vi "Main.vi"() -> ()   [LabVIEW 2018]
doc: "Cet exemple de projet Mesure continue est basé sur le modèle Gestionnaire de messages dans une file d'attente.\n\nLa boucle de gestion d'événements génère des messages en fonction des actions sur l'interface utilisateur.\n\nLa boucle de gestion de messages traite les messages générés par la boucle de gestion d'événements ou par d'autres messages. Il y a aussi des sous-VIs de boucle de gestion de messages d'acquisition et d'enregistrement, ainsi qu'une boucle de mise à jour du graphe déroulant."
uses:
  Settings/Settings.ctl
  Acquisition/Hardware Configuration.ctl
  Acquisition/Signal Type.ctl
  Logging/Logging Configuration.ctl
  controls/UI Data.ctl
  controls/UI State.ctl
  support/Message Queue/Enqueue Message (Single).vi
  support/Message Queue/Enqueue Message (Array).vi
  <vilib>/Utility/error.llb/Error Cluster From Error Code.vi
  <vilib>/ErrorRing/Error Ring.xnode
  Acquisition/Acquisition.lvlib
  Logging/Logging.lvlib
  Settings/Settings.lvlib
  support/User Event - Stop/User Event - Stop.lvlib
  support/Message Queue/Message Queue.lvlib
  Settings/Settings Dialog.vi
panel:
  in  "Panneaux":enum32{"MAPA Tech"}(tab)
  out "Graphe d'intensité":dbl[][](graph)
  out "Booléen":bool
  out "Longueur d'onde":dbl
  out "Puissance":dbl
  out "Puissance prédite":dbl
  out "Longueur d'onde":dbl(knob) scale=550.0..2550.0
  out "Puissance prédite":dbl(knob) scale=0.0..10.0
  out "Puissance":dbl(knob) scale=0.0..10.0
  in  "Param status":bool
  out "Données":waveform(dbl)[](graph)
  out "État":string
  in  "Quitter":bool
  in  "Arrêter":bool
  in  "Démarrer":bool
  in  "Paramètres":bool
  # "MAPA Tech"
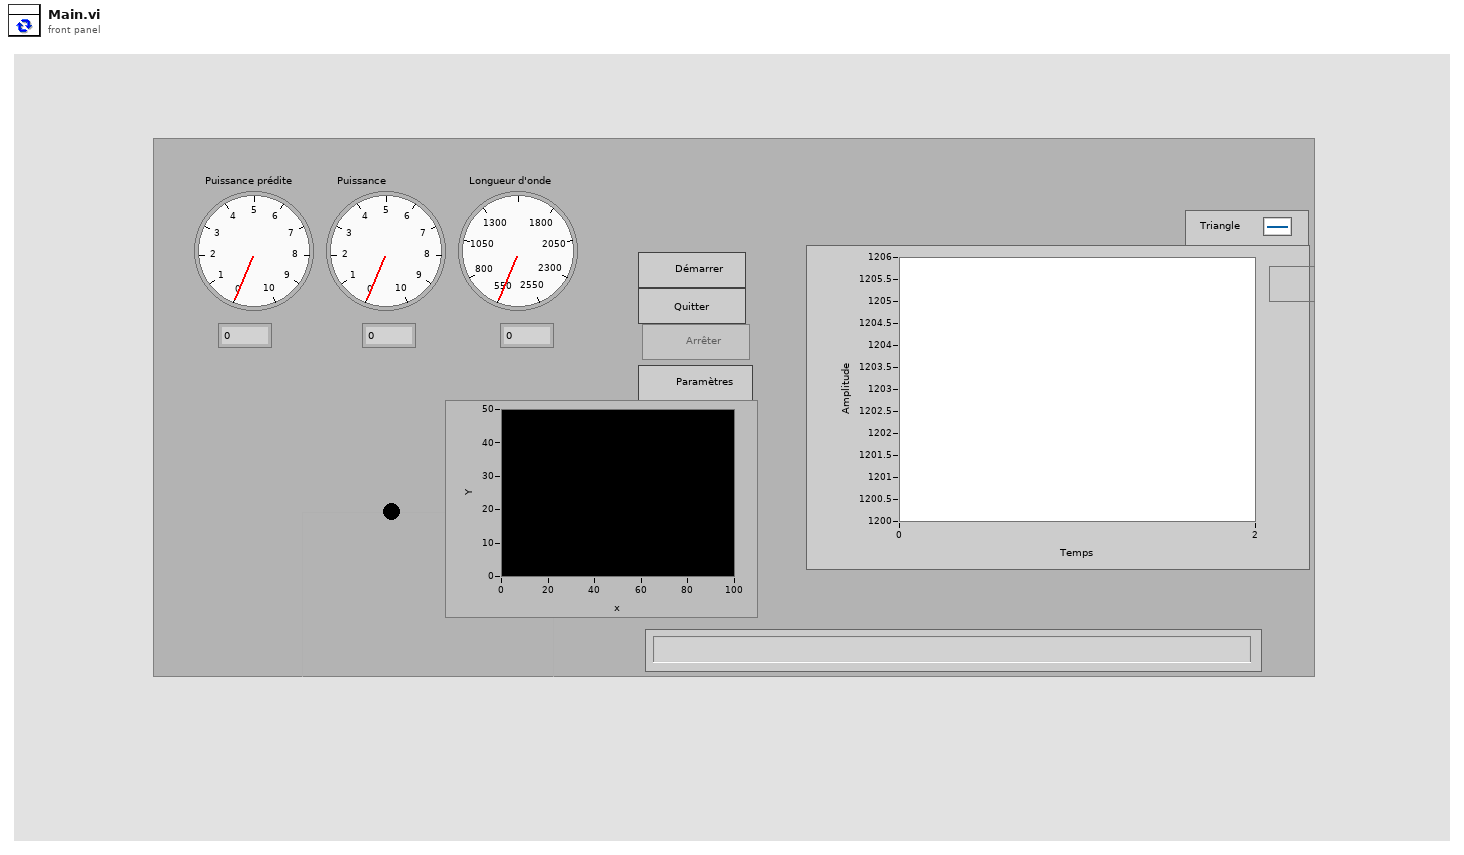
[diagram p1: front panel]
types:
  T1 = typedef "UI State.ctl" = enum16{"Idle", "Acquiring and Logging", "Waiting for Exit", "Waiting for Exit (Acq Stopped)", "Waiting for Exit (Log Stopped)", "Waiting for Stop", "Waiting for Stop (Acq Stopped)", "Waiting for Stop (Log Stopped)"}
  T2 = typedef "UI Data.ctl" = cluster{"Réf. de Démarrer":refnum<vi>, "Réf. d'Arrêter":refnum<vi>, "Réf. de Paramètres":refnum<vi>, "Réf. de Quitter":refnum<vi>, "Réf. d'état":refnum<vi>, "Réf. de données":refnum<vi>, "Ref. Moyennage sélectionneur":refnum<vi>, "Ref. Param status":refnum<vi>}
  T3 = typedef "Settings.lvlib/Settings.ctl" = cluster{"Configuration du matériel":T4, "Configuration de l'enregistrement":T6, "Commande numérique":dbl}
  T4 = typedef "Acquisition.lvlib/Hardware Configuration.ctl" = cluster{"Refnum de matériel <À remplacer>":string, "Type de signal <À remplacer>":T5, "Choix de la longueur d'onde":dbl, "Nom du périphérique":tag, "Choix mode":bool}
  T5 = typedef "Acquisition.lvlib/Signal Type.ctl" = enum16{"Sine Wave", "Square with Noise", "Signal triangulaire", "Simulation DAQ"}
  T6 = typedef "Logging.lvlib/Logging Configuration.ctl" = cluster{"Chemin de base du fichier journal":path, "Référence de fichier TDMS":refnum<k34>}
  T7 = cluster{"état":bool, "code":i32, "source":string}
  T8 = typedef "Message Queue.lvlib/All Message Queues.ctl" = cluster{"IU":refnum<queue>, "Acquisition":refnum<queue>, "Enregistrement":refnum<queue>}
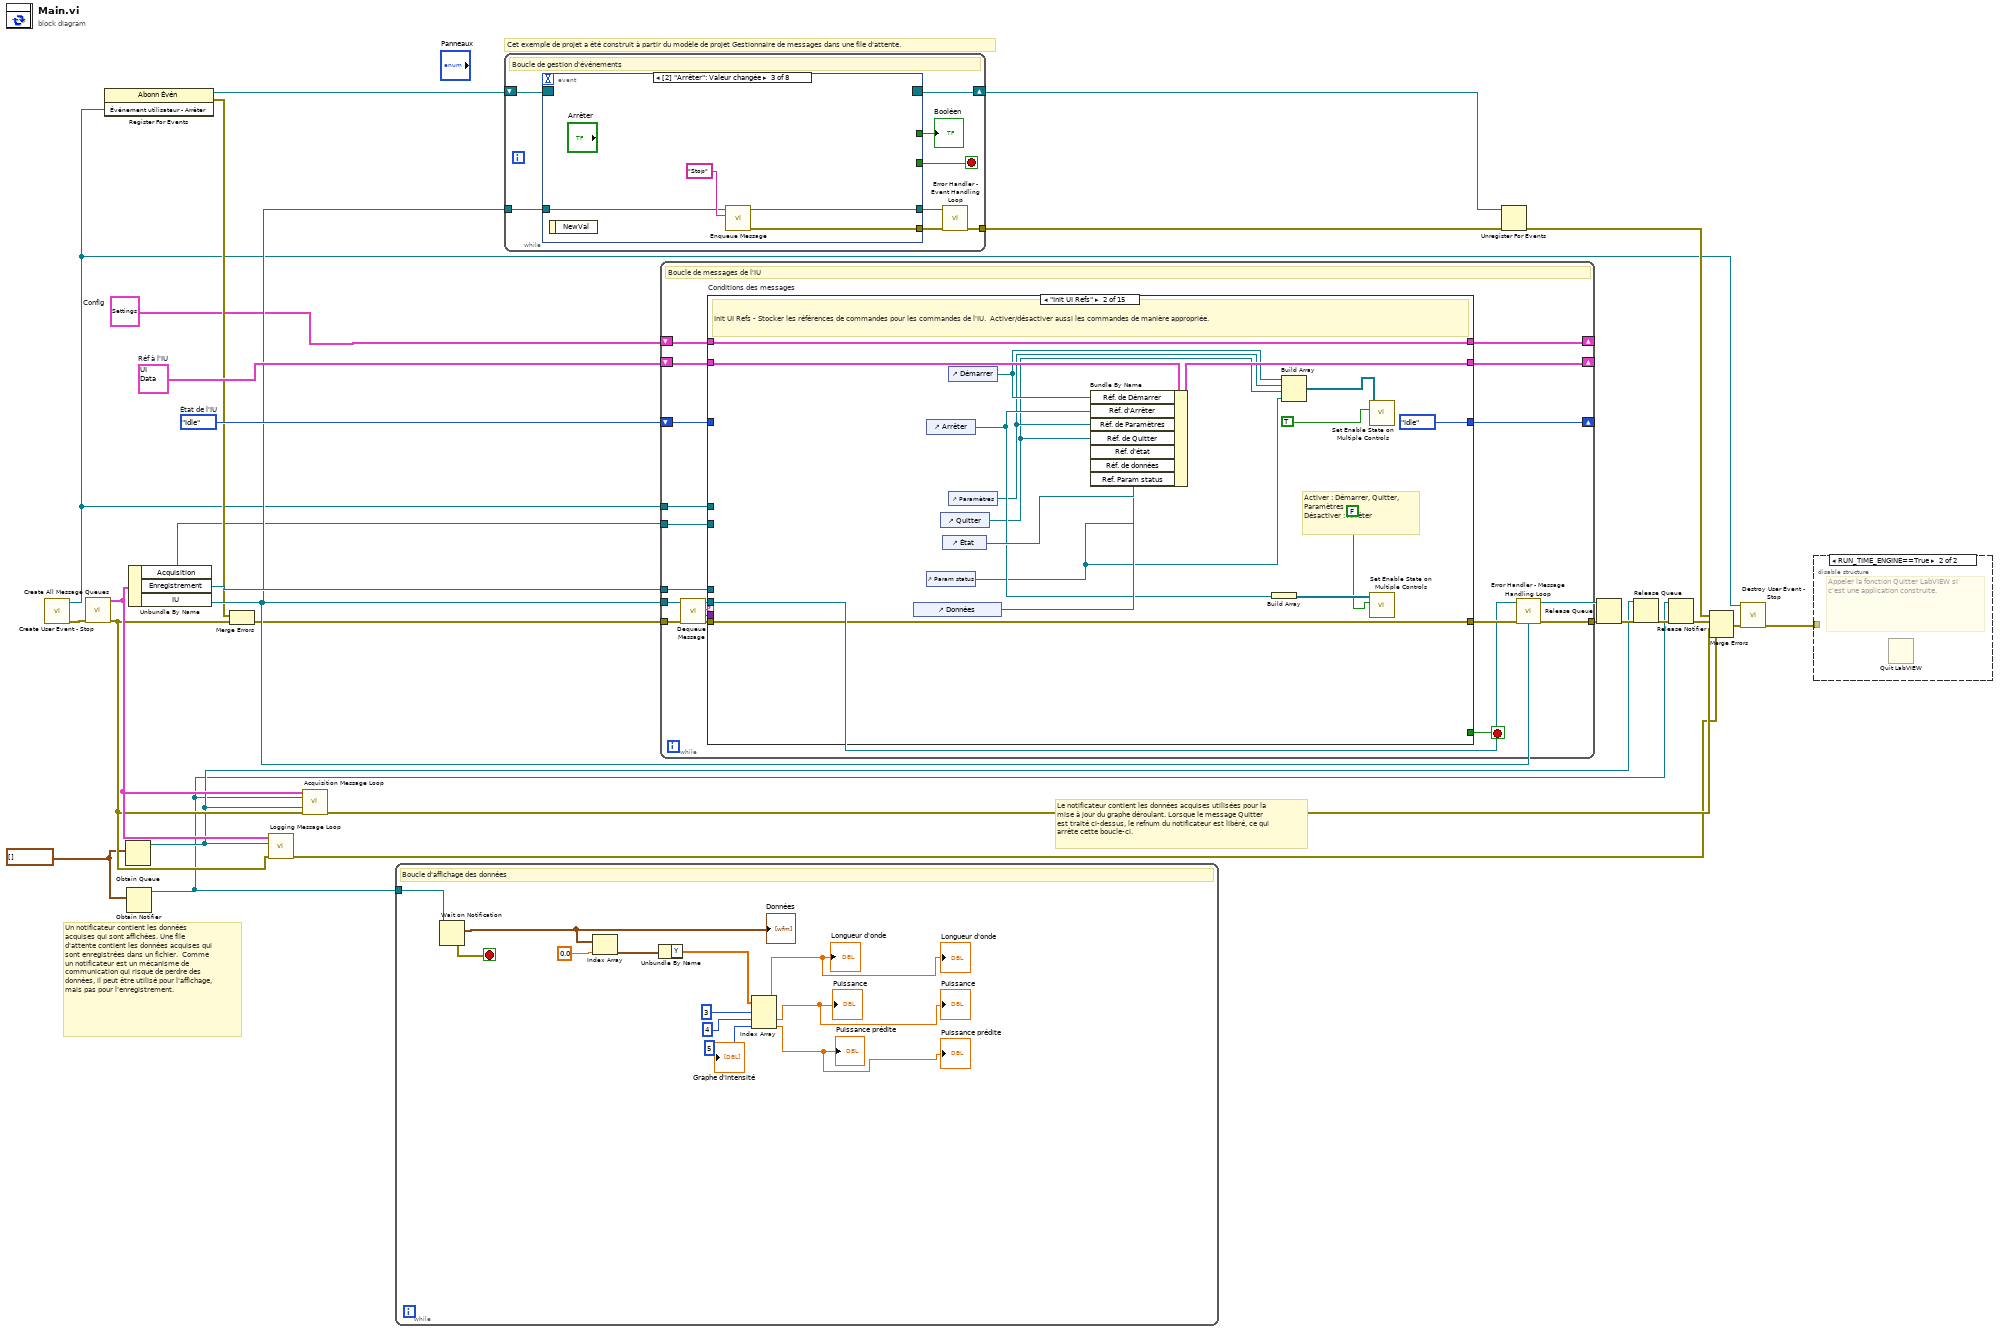
[diagram p0: block diagram]
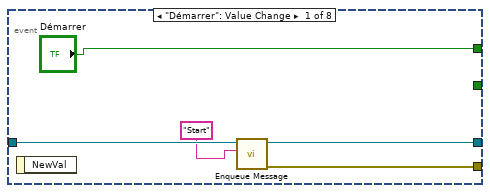
[diagram p3: hidden frame]
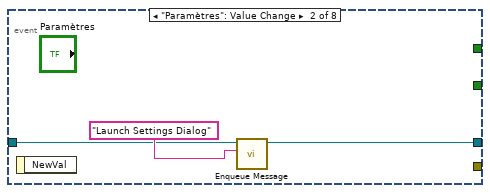
[diagram p4: hidden frame]
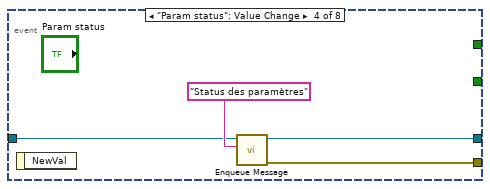
[diagram p5: hidden frame]
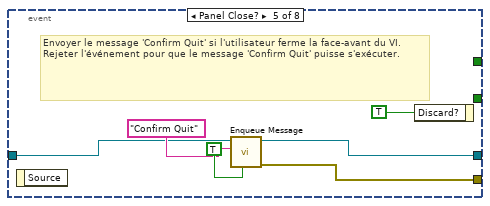
[diagram p6: hidden frame]
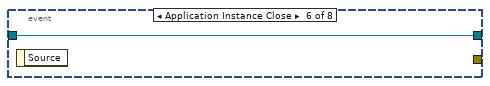
[diagram p7: hidden frame]
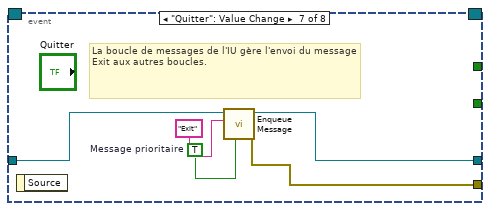
[diagram p8: hidden frame]
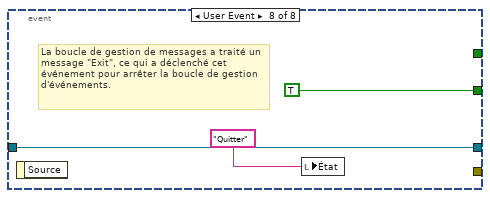
[diagram p9: hidden frame]
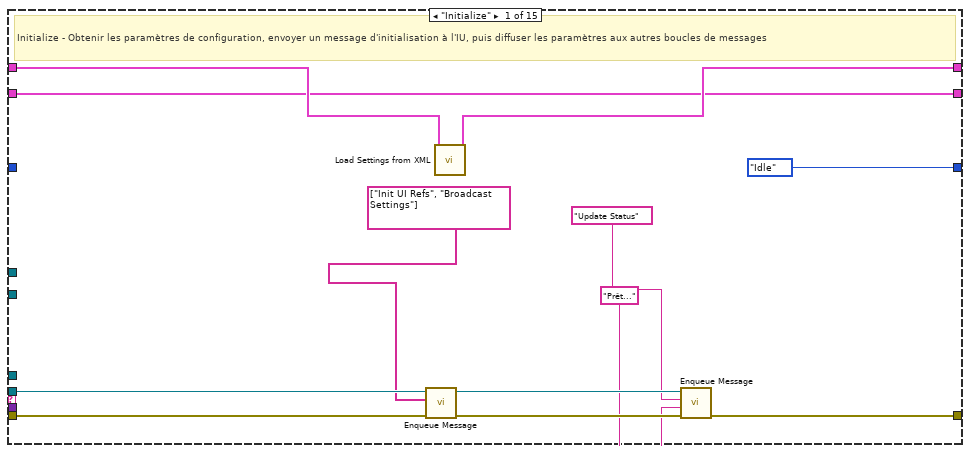
[diagram p10: hidden frame]
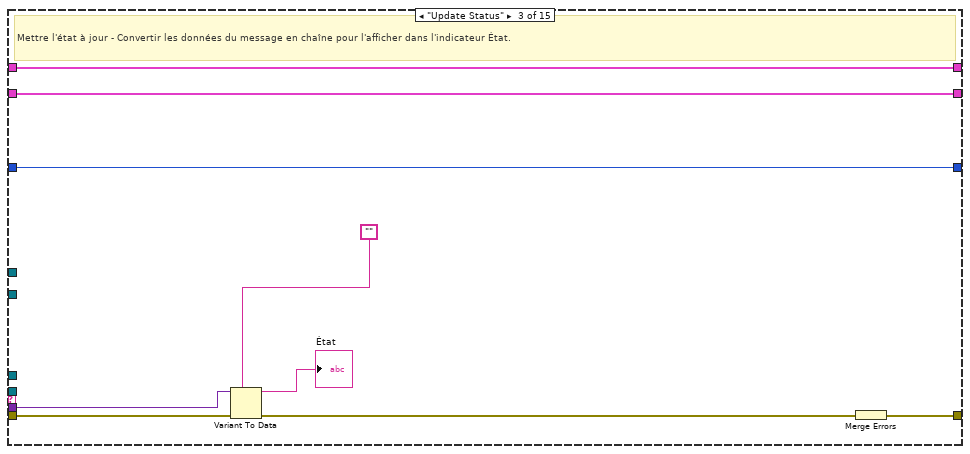
[diagram p11: hidden frame]
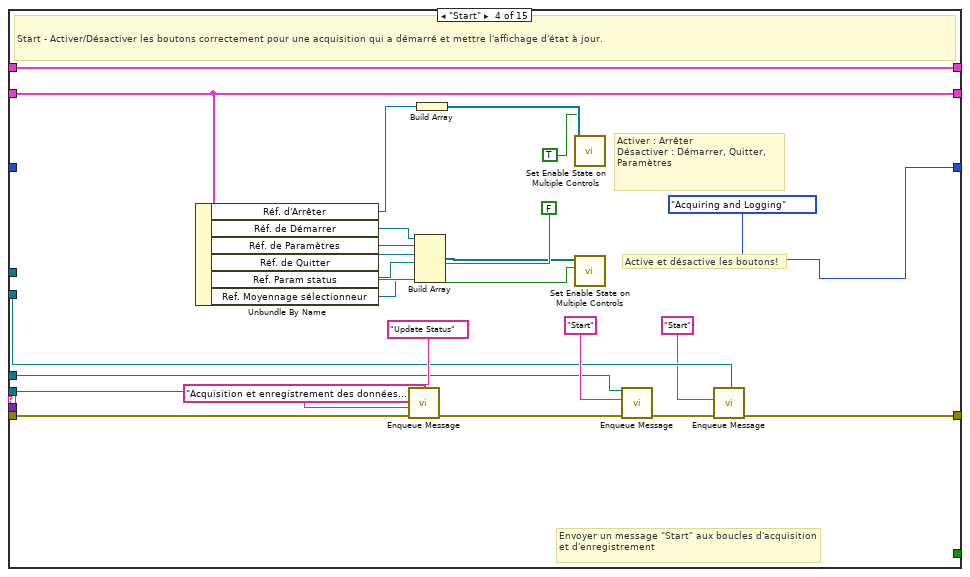
[diagram p12: hidden frame]
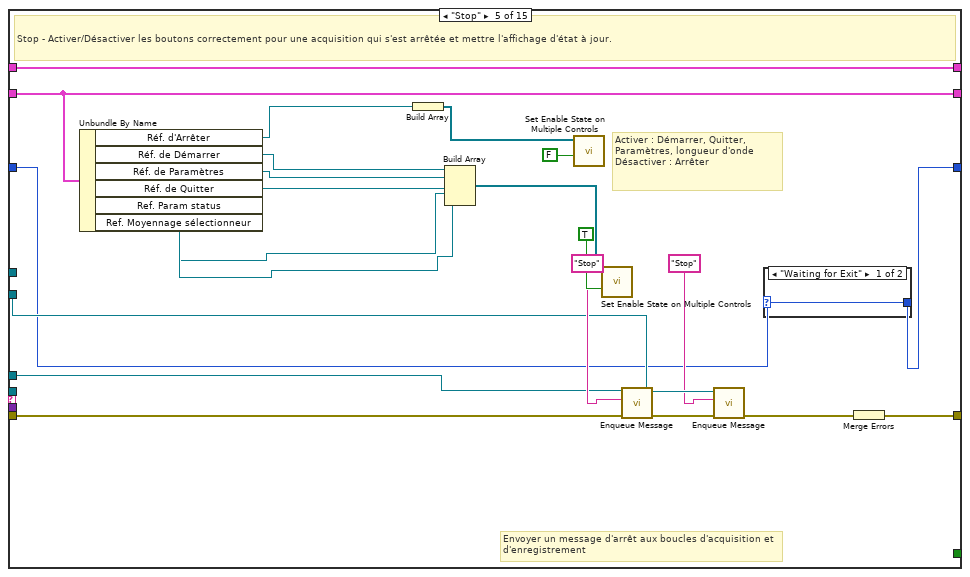
[diagram p13: hidden frame]
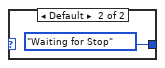
[diagram p14: hidden frame]
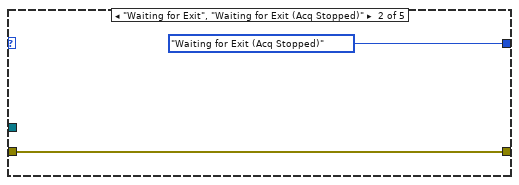
[diagram p16: hidden frame]
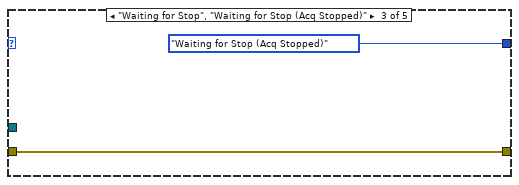
[diagram p17: hidden frame]
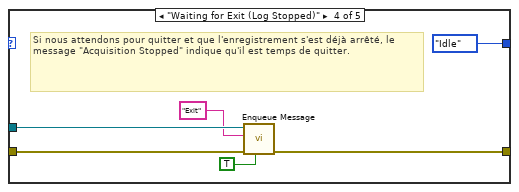
[diagram p18: hidden frame]
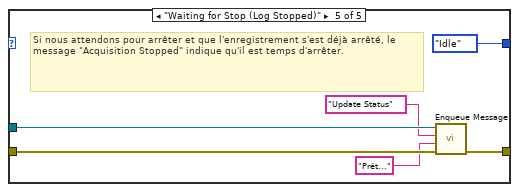
[diagram p19: hidden frame]
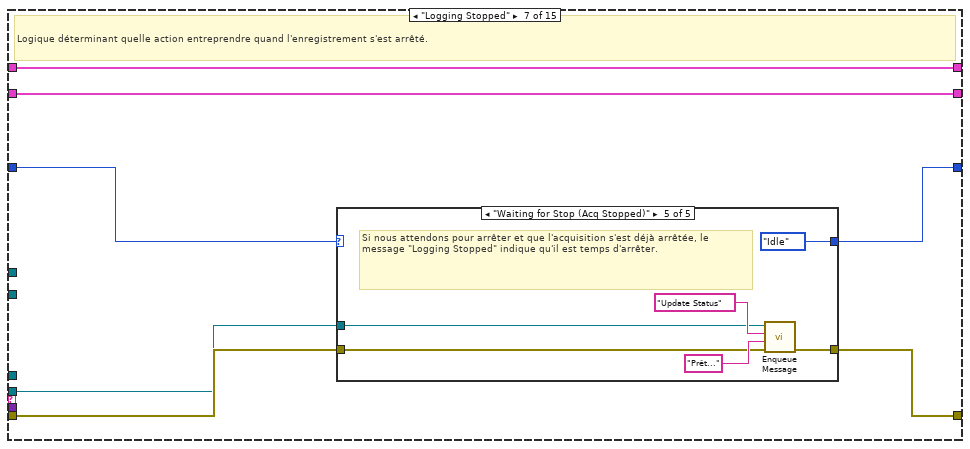
[diagram p20: hidden frame]
diagram:
  w16 = UI_State."Idle"  # État de l'IU
  w4 = waveform(dbl)[] []
  w18 = T2 {"Réf. de Démarrer"=refnum, "Réf. d'Arrêter"=refnum, "Réf. de Paramètres"=refnum, "Réf. de Quitter"=refnum, "Réf. d'état"=refnum, "Réf. de données"=refnum, "Ref. Moyennage sélectionneur"=refnum, "Ref. Param status"=refnum}  # Réf à l'IU
  w1 = T3 {"Configuration du matériel"={"Refnum de matériel <À remplacer>"="", "Type de signal <À remplacer>"=enum."Simulation DAQ", "Choix de la longueur d'onde"=500.0, "Nom du périphérique"="Dev1", "Choix mode"=FALSE}, "Configuration de l'enregistrement"={"Chemin de base du fichier journal"=path "", "Référence de fichier TDMS"=refnum}, "Commande numérique"=0.0}  # Config
  # "Cet exemple de projet a été construit à partir du modèle de projet Gestionnaire de messages dans une file d'attente."
  # "Un notificateur contient les données acquises qui sont affichées. Une file d'attente contient les données acquises qui sont enregistrées dans un fichier.  Comme un notificateur est un mécanisme de communication qui risque de perdre des données, il peut être utilisé pour l'affichage, mais pas pour l'enregistrement."
  # "Le notificateur contient les données acquises utilisées pour la mise à jour du graphe déroulant. Lorsque le message Quitter est traité ci-dessus, le refnum du notificateur est libéré, ce qui arrête cette boucle-ci."
  n1 = call "Create User Event - Stop.vi"() -> ("error out"=w24:T7, "Événement utilisateur - Arrêter"=w5:refnum<user-event>)  [unwired: 10 in]
  n2 = call "Create All Message Queues.vi"("error in (no error)"=w24) -> ("error out"=w21:T7, "Files d'attente de messages en sortie"=w23:T8)  [unwired: 9 in]
  n3 = register-events(w5) -> (reference out=w9:refnum<event-registration>, error out=w7:errorcluster)  [unwired: 2 in]
  n4 = Obtain Queue(element data type=w4) -> (queue out=w3:refnum<queue>)  [unwired: 4 in, 2 out]
  n5 = Obtain Notifier(notification data type=w4) -> (notifier out=w2:refnum<notifier>)  [unwired: 3 in, 2 out]
  n6 = Unbundle By Name(w23) -> ("Acquisition"=w6:refnum<queue>, "Enregistrement"=w17:refnum<queue>, "IU"=w14:refnum<queue>)
  n7 = Merge Errors(w7, w21) -> (w8:errorcluster)
  n8 = call "Logging Message Loop.vi"("error in (no error)"=w21, "File d'attente de données"=w3, "Files d'attente de messages"=w23) -> ("error out"=w22:T7)  [unwired: 8 in]
  n9 = call "Acquisition Message Loop.vi"("Files d'attente de messages"=w23, "Notificateur de données"=w2, "File d'attente de données"=w3, "error in (no error)"=w21) -> ("error out"=w25:T7)  [unwired: 11 in]
  n10 = while "Data Display Loop" {
    tunnel: w2 -> [w38]
    stop <- w39 stop-if-true
    # "Boucle d'affichage des données"
    n11 = Wait on Notification(notifier=w38) -> (notification=w36:waveform(dbl)[], error out=w39:errorcluster)  [unwired: 3 in, 2 out]
    "Données" <- w36
    n12 = Index Array(array=w36, index=0.0) -> (element=w35:waveform(dbl))
    n13 = Unbundle By Name(w35) -> ("Y"=w34:dbl[])
    n14 = Index Array(array=w34, index #1=3, index #2=4, index #3=5 ("indice")) -> (element #1=→"Longueur d'onde" →"Longueur d'onde":dbl, element #2=→"Puissance" →"Puissance":dbl, element #3=→"Puissance prédite" →"Puissance prédite":dbl)
  }
  n15 = while {
    tunnel: w14 -> [w46]
    tunnel: [w43] -> w26
    shift-right: [w45] -> w19
    shift-left: w9 -> [w47]
    stop <- w44 stop-if-true
    # "Boucle de gestion d'événements"
    n16 = event shown="[2] \"Arrêter\": Valeur changée" {
      selector: w47 -> [_ _ _ _ _ _ _ _]
      dyn-events: [_ _ _ _ _ _ _ _] -> w45
      timeout: _ -> [_ _ _ _ _ _ _ _]
      tunnel: [_ _ _ _ _ _ _ TRUE ("Discard?")] -> w44
      tunnel: w46 -> [w52 w54 w58 w62 w67 w70 w72 w76]
      tunnel: [w50 _ w57 w61 w65 _ w75 _] -> w42
      tunnel: [w49 w53 w56 w60 w66 w70 w71 w76] -> w41
      tunnel: ["Démarrer" _ _ _ _ _ _ _] -> w40
      event "Démarrer": Value Change {
        n17 = event-data() -> ()  [unwired: 1 in, 1 out]
        n18 = call-poly "Enqueue Message.vi"("Message"="Start", "File d'attente de messages"=w52) -> ("error out"=w50:T7, "File d'attente de message dup."=w49:refnum<queue>)  [unwired: 8 in]
      }
      event "Paramètres": Value Change {
        n19 = event-data() -> ()  [unwired: 1 in, 1 out]
        n20 = call-poly "Enqueue Message.vi"("Message"="Launch Settings Dialog", "File d'attente de messages"=w54) -> ("File d'attente de message dup."=w53:refnum<queue>)  [unwired: 8 in, 1 out]
      }
      event "Arrêter": Value Change {
        n21 = event-data() -> ()  [unwired: 1 in, 1 out]
        n22 = call-poly "Enqueue Message.vi"("Message"="Stop", "File d'attente de messages"=w58) -> ("error out"=w57:T7, "File d'attente de message dup."=w56:refnum<queue>)  [unwired: 8 in]
      }
      event "Param status": Value Change {
        n23 = event-data() -> ()  [unwired: 1 in, 1 out]
        n24 = call-poly "Enqueue Message.vi"("Message"="Status des paramètres", "File d'attente de messages"=w62) -> ("error out"=w61:T7, "File d'attente de message dup."=w60:refnum<queue>)  [unwired: 8 in]
      }
      event Panel Close? {
        # "Envoyer le message 'Confirm Quit' si l'utilisateur ferme la face-avant du VI. Rejeter l'événement pour que le message 'Confirm Quit' puisse s'exécuter."
        n25 = event-data() -> ()  [unwired: 1 in, 1 out]
        n26 = call-poly "Enqueue Message.vi"("Message prioritaire ? (F)"=TRUE ("Priority Message? (F)"), "Message"="Confirm Quit", "File d'attente de messages"=w67) -> ("error out"=w65:T7, "File d'attente de message dup."=w66:refnum<queue>)  [unwired: 7 in]
        n27 = event-data ("Event Filter Node")("Discard?"=TRUE) -> ()  [unwired: 1 in, 1 out]
      }
      event Application Instance Close {
        n28 = event-data() -> ()  [unwired: 1 in, 1 out]
      }
      event "Quitter": Value Change {
        w73 = TRUE  # Message prioritaire
        # "La boucle de messages de l'IU gère l'envoi du message Exit aux autres boucles."
        n29 = event-data() -> ()  [unwired: 1 in, 1 out]
        n30 = call-poly "Enqueue Message.vi"("Message prioritaire ? (F)"=w73, "Message"="Exit", "File d'attente de messages"=w72) -> ("error out"=w75:T7, "File d'attente de message dup."=w71:refnum<queue>)  [unwired: 7 in]
      }
      event User Event {
        # "La boucle de gestion de messages a traité un message \"Exit\", ce qui a déclenché cet événement pour arrêter la boucle de gestion d'événements."
        n31 = event-data() -> ()  [unwired: 1 in, 1 out]
        n32 = local write "État"("Quitter" ("Exit String")) -> ()
      }
    }
    "Booléen" <- w40
    n33 = call "Error Handler - Event Handling Loop.vi"("error in (no error)"=w42, "File d'attente de messages"=w41) -> ("erreur en entrée dup."=w43:T7)  [unwired: 8 in, 1 out]
  }
  n34 = while {
    tunnel: w14 -> [w90]
    tunnel: w5 -> [w95]
    shift-right: [w89] -> _
    shift-left: w1 -> [w88]
    shift-right: [w86] -> _
    shift-left: w18 -> [w87]
    tunnel: w6 -> [w85]
    tunnel: w17 -> [w84]
    shift-right: [w79] -> _
    shift-left: w16 -> [w80]
    tunnel: w8 -> [w94]
    tunnel: [w83] -> w27
    stop <- w96 stop-if-true
    # "Boucle de messages de l'IU"
    n35 = call "Dequeue Message.vi"("error in (no error)"=w94, "File d'attente de messages"=w90) -> ("error out"=w93:T7, "Données de message"=w91:variant, "Message"=w92:string, "File d'attente de message dup."=w81:refnum<queue>)  [unwired: 6 in]
    n36 = case "Conditions des messages" shown="\"Init UI Refs\"" w92 {
      selector: w92 -> [_ _ _ _ _ _ _ _ _ _ _ _ _ _ w334]
      tunnel: w81 -> [w100 _ _ w157 _ w184 w209 _ w249 _ w270 _ _ w321 _]
      tunnel: w93 -> [w99 w124 w132 w156 w178 w185 w210 w237 w251 w258 w269 w298 w315 w325 _]
      tunnel: [w104 w124 w133 w143 w179 w182 w207 w243 w244 w261 w268 w308 w314 w324 w333] -> w82
      tunnel: [_ _ _ _ _ _ _ _ _ _ _ TRUE _ _ _] -> w96
      tunnel: w91 -> [_ _ w131 _ _ _ _ _ _ w262 _ w296 _ _ _]
      tunnel: w95 -> [_ _ _ _ _ _ _ _ _ _ _ w309 _ _ _]
      tunnel: [w107 w123 w127 w155 w177 w188 w213 w241 w248 w266 w273 w307 w313 w319 w337] -> w89
      tunnel: w88 -> [w108 w123 w127 w155 w177 w188 w213 w241 w252 w266 w273 w307 w313 w319 w337]
      tunnel: w87 -> [w101 w122 w126 w152 w176 w187 w212 w236 w246 w265 w272 w306 w312 w323 w336]
      tunnel: [w101 w119 w126 w152 w176 w187 w212 w236 w246 w265 w272 w306 w312 w323 w336] -> w86
      tunnel: w85 -> [_ _ _ w142 w169 _ _ w235 _ _ _ w305 _ _ _]
      tunnel: w84 -> [_ _ _ w145 w172 _ _ w232 _ _ _ w304 _ _ _]
      tunnel: w80 -> [_ _ w125 _ w166 w186 w211 w234 w245 w260 w271 _ w311 _ w335]
      tunnel: [UI_State."Idle" ("UI State") UI_State."Idle" ("UI State") w125 UI_State."Acquiring and Logging" ("UI State") w167 w183 w208 w234 w245 w260 w267 UI_State."Idle" ("UI State") w311 UI_State."Acquiring and Logging" ("UI State") w335] -> w79
      frame "Initialize" {
        # "Initialize - Obtenir les paramètres de configuration, envoyer un message d'initialisation à l'IU, puis diffuser les paramètres aux autres boucles de messages"
        n37 = call-poly "Enqueue Message.vi"("error in (no error)"=w99, "Tableau de messages"=string[] ["Init UI Refs", "Broadcast Settings"], "File d'attente de messages"=w100) -> ("error out"=w106:T7, "File d'attente de message dup."=w105:refnum<queue>)  [unwired: 7 in]
        n38 = call "Load Settings from XML.vi"("Paramètres en entrée"=w108) -> ("Paramètres en sortie"=w107:T3)  [unwired: 9 in, 1 out]
        n39 = call-poly "Enqueue Message.vi"("error in (no error)"=w106, "Données de message"="Prêt..." ("Ready..."), "Message"="Update Status", "File d'attente de messages"=w105) -> ("error out"=w104:T7)  [unwired: 6 in, 1 out]
      }
      frame "Init UI Refs" {
        # "Activer : Démarrer, Quitter, Paramètres\nDésactiver : Arrêter"
        # "Init UI Refs - Stocker les références de commandes pour les commandes de l'IU.  Activer/désactiver aussi les commandes de manière appropriée."
        n40 = control-ref of="Données"() -> (w120:refnum<vi>)
        n41 = control-ref of="Param status"() -> (w109:refnum<vi>)
        n42 = control-ref of="Arrêter"() -> (w114:refnum<vi>)
        n43 = control-ref of="Quitter"() -> (w111:refnum<vi>)
        n44 = control-ref of="État"() -> (w121:refnum<vi>)
        n45 = control-ref of="Démarrer"() -> (w113:refnum<vi>)
        n46 = control-ref of="Paramètres"() -> (w112:refnum<vi>)
        n47 = Bundle By Name(cluster=w122, "Réf. de Démarrer"=w113, "Réf. d'Arrêter"=w114, "Réf. de Paramètres"=w112, "Réf. de Quitter"=w111, "Réf. d'état"=w121, "Réf. de données"=w120, "Ref. Param status"=w109) -> (w119:T2)
        n48 = Build Array(w114) -> (w116:refnum<vi>[])
        n49 = Build Array(w113, w112, w111, w109) -> (w117:refnum<vi>[])
        n50 = call "Set Enable State on Multiple Controls.vi"("Activé ?"=TRUE ("Enable?"), "Commandes"=w117) -> ()  [unwired: 10 in]
        n51 = call "Set Enable State on Multiple Controls.vi"("Activé ?"=FALSE ("Enable?"), "Commandes"=w116) -> ()  [unwired: 10 in]
      }
      frame "Update Status" {
        # "Mettre l'état à jour - Convertir les données du message en chaîne pour l'afficher dans l'indicateur État."
        n52 = Variant To Data(error in=w132, type="" ("Empty String Constant"), Variant=w131) -> (data=→"État":string, error out=w129:errorcluster)
        n53 = Merge Errors(w129) -> (w133:errorcluster)
      }
      frame "Start" {
        # "Active et désactive les boutons!"
        # "Envoyer un message \"Start\" aux boucles d'acquisition et d'enregistrement"
        # "Activer : Arrêter\nDésactiver : Démarrer, Quitter, Paramètres"
        # "Start - Activer/Désactiver les boutons correctement pour une acquisition qui a démarré et mettre l'affichage d'état à jour."
        n54 = Unbundle By Name(w152) -> ("Réf. d'Arrêter"=w134:refnum<vi>, "Réf. de Démarrer"=w135:refnum<vi>, "Réf. de Paramètres"=w136:refnum<vi>, "Réf. de Quitter"=w139:refnum<vi>, "Ref. Param status"=w138:refnum<vi>, "Ref. Moyennage sélectionneur"=w137:refnum<vi>)
        n55 = call-poly "Enqueue Message.vi"("error in (no error)"=w156, "Données de message"="Acquisition et enregistrement des données..." ("Acquiring and Logging..."), "Message"="Update Status", "File d'attente de messages"=w157) -> ("error out"=w147:T7)  [unwired: 6 in, 1 out]
        n56 = Build Array(w135, w136, w136, w139, w138, w137) -> (w150:refnum<vi>[])
        n57 = Build Array(w134) -> (w149:refnum<vi>[])
        n58 = call "Set Enable State on Multiple Controls.vi"("Activé ?"=TRUE ("Enable?"), "Commandes"=w149) -> ()  [unwired: 10 in]
        n59 = call "Set Enable State on Multiple Controls.vi"("Activé ?"=FALSE ("Enable?"), "Commandes"=w150) -> ()  [unwired: 10 in]
        n60 = call-poly "Enqueue Message.vi"("error in (no error)"=w147, "Message"="Start", "File d'attente de messages"=w145) -> ("error out"=w144:T7)  [unwired: 7 in, 1 out]
        n61 = call-poly "Enqueue Message.vi"("error in (no error)"=w144, "Message"="Start", "File d'attente de messages"=w142) -> ("error out"=w143:T7)  [unwired: 7 in, 1 out]
      }
      frame "Stop" {
        # "Envoyer un message d'arrêt aux boucles d'acquisition et d'enregistrement"
        # "Activer : Démarrer, Quitter, Paramètres, longueur d'onde\nDésactiver : Arrêter"
        # "Stop - Activer/Désactiver les boutons correctement pour une acquisition qui s'est arrêtée et mettre l'affichage d'état à jour."
        n62 = Unbundle By Name(w176) -> ("Réf. d'Arrêter"=w158:refnum<vi>, "Réf. de Démarrer"=w159:refnum<vi>, "Réf. de Paramètres"=w160:refnum<vi>, "Réf. de Quitter"=w161:refnum<vi>, "Ref. Param status"=w162:refnum<vi>, "Ref. Moyennage sélectionneur"=w163:refnum<vi>)
        n63 = Build Array(w158) -> (w164:refnum<vi>[])
        n64 = Build Array(w159, w160, w161, w162, w163) -> (w165:refnum<vi>[])
        n65 = call "Set Enable State on Multiple Controls.vi"("Activé ?"=FALSE ("Enable?"), "Commandes"=w164) -> ()  [unwired: 10 in]
        n66 = call "Set Enable State on Multiple Controls.vi"("Activé ?"=TRUE ("Enable?"), "Commandes"=w165) -> ()  [unwired: 10 in]
        n67 = call-poly "Enqueue Message.vi"("error in (no error)"=w178, "Message"="Stop", "File d'attente de messages"=w172) -> ("error out"=w171:T7)  [unwired: 7 in, 1 out]
        n68 = call-poly "Enqueue Message.vi"("error in (no error)"=w171, "Message"="Stop", "File d'attente de messages"=w169) -> ("error out"=w170:T7)  [unwired: 7 in, 1 out]
        n69 = case shown="\"Waiting for Exit\"" w166 {
          selector: w166 -> [w180 _]
          tunnel: [w180 UI_State."Waiting for Stop" ("UI State")] -> w167
          frame "Waiting for Exit" {
          }
          frame Default {
          }
        }
        n70 = Merge Errors(w170) -> (w179:errorcluster)
      }
      frame "Acquisition Stopped" {
        # "Logique déterminant quelle action entreprendre quand l'acquisition s'est arrêtée."
        n71 = case shown="Par défaut" w186 {
          selector: w186 -> [w190 _ _ _ _]
          tunnel: w185 -> [w189 w192 w194 w200 w206]
          tunnel: w184 -> [_ _ _ w198 w203]
          tunnel: [w190 UI_State."Waiting for Exit (Acq Stopped)" ("UI State") UI_State."Waiting for Stop (Acq Stopped)" ("UI State") UI_State."Idle" ("UI State") UI_State."Idle" ("UI State")] -> w183
          tunnel: [w189 w192 w194 w199 w204] -> w182
          frame Default {
          }
          frame "Waiting for Exit", "Waiting for Exit (Acq Stopped)" {
          }
          frame "Waiting for Stop", "Waiting for Stop (Acq Stopped)" {
          }
          frame "Waiting for Exit (Log Stopped)" {
            # "Si nous attendons pour quitter et que l'enregistrement s'est déjà arrêté, le message \"Acquisition Stopped\" indique qu'il est temps de quitter."
            n72 = call-poly "Enqueue Message.vi"("Message prioritaire ? (F)"=TRUE ("Priority Message? (F)"), "error in (no error)"=w200, "Message"="Exit", "File d'attente de messages"=w198) -> ("error out"=w199:T7)  [unwired: 6 in, 1 out]
          }
          frame "Waiting for Stop (Log Stopped)" {
            # "Si nous attendons pour arrêter et que l'enregistrement s'est déjà arrêté, le message \"Acquisition Stopped\" indique qu'il est temps d'arrêter."
            n73 = call-poly "Enqueue Message.vi"("error in (no error)"=w206, "Données de message"="Prêt..." ("Ready..."), "Message"="Update Status", "File d'attente de messages"=w203) -> ("error out"=w204:T7)  [unwired: 6 in, 1 out]
          }
        }
      }
      frame "Logging Stopped" {
        # "Logique déterminant quelle action entreprendre quand l'enregistrement s'est arrêté."
        n74 = case shown="\"Waiting for Stop (Acq Stopped)\"" w211 {
          selector: w211 -> [w215 _ _ _ _]
          tunnel: w210 -> [w214 w217 w219 w225 w228]
          tunnel: w209 -> [_ _ _ w223 w227]
          tunnel: [w215 UI_State."Waiting for Exit (Log Stopped)" ("UI State") UI_State."Waiting for Stop (Log Stopped)" ("UI State") UI_State."Idle" ("UI State") UI_State."Idle" ("UI State")] -> w208
          tunnel: [w214 w217 w219 w224 w226] -> w207
          frame Default {
          }
          frame "Waiting for Exit", "Waiting for Exit (Log Stopped)" {
          }
          frame "Waiting for Stop", "Waiting for Stop (Log Stopped)" {
          }
          frame "Waiting for Exit (Acq Stopped)" {
            # "Si nous attendons pour quitter et que l'acquisition s'est déjà arrêtée, le message \"Logging Stopped\" indique qu'il est temps de quitter."
            n75 = call-poly "Enqueue Message.vi"("Message prioritaire ? (F)"=TRUE ("Priority Message? (F)"), "error in (no error)"=w225, "Message"="Exit", "File d'attente de messages"=w223) -> ("error out"=w224:T7)  [unwired: 6 in, 1 out]
          }
          frame "Waiting for Stop (Acq Stopped)" {
            # "Si nous attendons pour arrêter et que l'acquisition s'est déjà arrêtée, le message \"Logging Stopped\" indique qu'il est temps d'arrêter."
            n76 = call-poly "Enqueue Message.vi"("error in (no error)"=w228, "Données de message"="Prêt..." ("Ready..."), "Message"="Update Status", "File d'attente de messages"=w227) -> ("error out"=w226:T7)  [unwired: 6 in, 1 out]
          }
        }
      }
      frame "Broadcast settings" {
        w233 = "Update Settings" ("Message")
        # "Broadcast settings - Envoyer le message 'Update Settings' aux boucles de messages d'enregistrement et d'acquisition."
        n77 = Unbundle By Name(w241) -> ("Configuration du matériel"=w240:T4, "Configuration de l'enregistrement"=w239:T6)
        n78 = call-poly "Enqueue Message.vi"("Données de message"=w240, "Message"=w233, "File d'attente de messages"=w235) -> ("error out"=w242:T7)  [unwired: 7 in, 1 out]
        n79 = call-poly "Enqueue Message.vi"("error in (no error)"=w242, "Données de message"=w239, "Message"=w233, "File d'attente de messages"=w232) -> ("error out"=w238:T7)  [unwired: 6 in, 1 out]
        n80 = Merge Errors(w238, w237) -> (w243:errorcluster)
      }
      frame "Launch Settings Dialog" {
        # "Launch Settings Dialog - Lancer la boîte de dialogue Paramètres quand l'utilisateur clique sur le bouton Paramètres."
        n81 = call-by-ref "?"("error in (no error)"=w251, "Paramètres en entrée"=w252) -> ("error out"=w247:T7, "Annulation ?"=w250:bool, "Paramètres en sortie"=w248:T3)  [unwired: 8 in, 3 out]
        n82 = case shown="Faux" w250 {
          tunnel: w249 -> [w256 _]
          tunnel: w247 -> [w255 w257]
          tunnel: [w254 w257] -> w244
          frame False {
            n83 = call-poly "Enqueue Message.vi"("error in (no error)"=w255, "Message"="Broadcast Settings", "File d'attente de messages"=w256) -> ("error out"=w254:T7)  [unwired: 7 in, 1 out]
          }
          frame True {
          }
        }
      }
      frame "Error" {
        # "Error - Afficher une boîte de dialogue d'erreur. Ce message est envoyé par les VIs \"Error Handler\" à la fin de l'exécution de chaque boucle de cette application."
        n84 = Variant To Data(error in=w258, type=errorcluster {"status"=FALSE, "code"=0, "source"=""} ("error constant"), Variant=w262) -> (data=w259:errorcluster, error out=w263:errorcluster)
        n85 = call <vilib>:"Simple Error Handler.vi"("error in (no error)"=w259) -> ()  [unwired: 4 in, 5 out]
        n86 = Merge Errors(w263) -> (w261:errorcluster)
      }
      frame "Confirm Quit" {
        # "Confirm Quit - Message qui confirme si l'utilisateur voulait vraiment quitter l'application."
        n87 = case shown="\"Acquiring and Logging\"" w271 {
          tunnel: w270 -> [w279 w283]
          tunnel: w269 -> [w278 w282]
          tunnel: [w277 w281] -> w268
          tunnel: [UI_State."Idle" ("UI State") w280] -> w267
          frame Default {
            # "Si 'Confirm Quit' survient alors que le système est inactif, le message de confirmation est inutile."
            n88 = call-poly "Enqueue Message.vi"("Message prioritaire ? (F)"=TRUE ("Priority Message? (F)"), "error in (no error)"=w278, "Message"="Exit", "File d'attente de messages"=w279) -> ("error out"=w277:T7)  [unwired: 6 in, 1 out]
          }
          frame "Acquiring and Logging" {
            n89 = Two Button Dialog(message="Voulez-vous vraiment quitter en cours d'acquisition ?" ("Confirm Quit Message"), 1:"Non" ("No"), 2:"Oui" ("Yes")) -> (T button?=w284:bool)
            n90 = case shown="Vrai" w284 {
              tunnel: w283 -> [_ w293]
              tunnel: w282 -> [w289 w294]
              tunnel: [w289 w292] -> w281
              tunnel: [UI_State."Acquiring and Logging" ("UI State") UI_State."Waiting for Exit" ("UI State")] -> w280
              frame False {
                # "L'utilisateur ne voulait pas quitter."
              }
              frame True {
                n91 = call-poly "Enqueue Message.vi"("error in (no error)"=w294, "Message"="Stop", "File d'attente de messages"=w293) -> ("error out"=w292:T7)  [unwired: 7 in, 1 out]
              }
            }
          }
        }
      }
      frame "Exit" {
        w300 = TRUE ("Priority Message? (F)")
        w301 = "Exit" ("Message")
        # "Afficher une boîte de dialogue d'erreur si 'Exit' a été appelé suite à une erreur."
        # "Arrêter le VI"
        # "Exit - Envoyer des messages Exit aux boucles d'acquisition et d'enregistrerment, et déclencher l'événement utilisateur pour arrêter la boucle de gestion d'événements."
        n92 = Variant To Data(type=errorcluster {"status"=FALSE, "code"=0, "source"=""} ("error constant"), Variant=w296) -> (data=w295:errorcluster)  [unwired: 1 in, 1 out]
        n93 = call <vilib>:"Simple Error Handler.vi"("error in (no error)"=w295) -> ()  [unwired: 4 in, 5 out]
        n94 = call-poly "Enqueue Message.vi"("Message prioritaire ? (F)"=w300, "error in (no error)"=w298, "Message"=w301, "File d'attente de messages"=w305) -> ("error out"=w302:T7)  [unwired: 6 in, 1 out]
        n95 = call-poly "Enqueue Message.vi"("Message prioritaire ? (F)"=w300, "error in (no error)"=w302, "Message"=w301, "File d'attente de messages"=w304) -> ("error out"=w299:T7)  [unwired: 6 in, 1 out]
        n96 = call "Fire User Event - Stop.vi"("error in (no error)"=w299, "Événement utilisateur - Arrêt"=w309) -> ("error out"=w308:T7)  [unwired: 9 in]
      }
      frame "---Copy This Frame---" {
        # "Dupliquez cette étape pour créer de nouveaux messages.  Changez ce commentaire dans l'étape dupliquée pour décrire ce message."
        n97 = Merge Errors(w315) -> (w314:errorcluster)
      }
      frame "Status des paramètres" {
        # "Dupliquez cette étape pour créer de nouveaux messages.  Changez ce commentaire dans l'étape dupliquée pour décrire ce message."
        n98 = Unbundle By Name(w319) -> ("Configuration du matériel.Choix mode"=w318:bool, "Configuration du matériel.Choix de la longueur d'onde"=w317:dbl)
        n99 = case shown="Vrai" w318 {
          tunnel: [w326 w331] -> w316
          tunnel: w317 -> [_ w332]
          frame False {
            n100 = Concatenate Strings ("Concaténer des chaînes")("Status: Mode automatique") -> (w326:string)
          }
          frame True {
            n101 = Number To Decimal String(number=w332) -> (decimal integer string=w329:string)  [unwired: 1 in]
            n102 = Concatenate Strings ("Concaténer des chaînes")("Status: Mode manuel et la longueur d'onde sélectionnée est ", w329, " nm.") -> (w331:string)
          }
        }
        n103 = Merge Errors(w325) -> (w324:errorcluster)
        n104 = call-poly "Enqueue Message.vi"("Données de message"=w316, "Message"="Update Status", "File d'attente de messages"=w321) -> ()  [unwired: 7 in, 2 out]
      }
      frame Default {
        # "La condition 'Par défaut' ne s'exécute que s'il y a un message qui n'est défini dans aucune des autres conditions.  Renvoyer une erreur de programmation."
        n105 = xnode ("Error Ring")("paramètre 0"=w334) -> ("sortie d'erreur"=w333:errorcluster)
      }
    }
    n106 = call "Error Handler - Message Handling Loop.vi"("error in (no error)"=w82, "File d'attente de messages"=w81) -> ("erreur en entrée dup."=w83:T7)  [unwired: 8 in, 1 out]
  }
  n107 = Unregister For Events(event registration refnum=w19, error in=w26) -> (error out=w20:errorcluster)
  n108 = Release Queue(queue=w14, error in (no error)=w27) -> (error out=w12:errorcluster)  [unwired: 1 in, 2 out]
  n109 = Release Queue(queue=w3, error in (no error)=w12) -> (error out=w11:errorcluster)  [unwired: 1 in, 2 out]
  n110 = Release Notifier(notifier=w2, error in (no error)=w11) -> (error out=w10:errorcluster)  [unwired: 1 in, 2 out]
  n111 = Merge Errors(w20, w10, w25, w22) -> (w15:errorcluster)
  n112 = call "Destroy User Event - Stop.vi"("error in (no error)"=w15, "Événement utilisateur - Arrêt"=w5) -> ("error out"=w13:T7)  [unwired: 9 in]
  n113 = disable-structure "Conditional Disable Structure" shown="RUN_TIME_ENGINE==True" {
    disable-tunnel: w13 -> [_ _]
    frame condition #0 (active) {
    }
    frame condition #1 {
      # "Appeler la fonction Quitter LabVIEW si c'est une application construite."
      n114 = Quit LabVIEW() -> ()  [unwired: 1 in]
    }
  }
